vi "2_06.vi"() -> ()   [LabVIEW 2018]
uses:
  <vilib>/sound2/lvsound2.llb/Sound Data Format.ctl
  <vilib>/sound2/lvsound2.llb/Sound Input Read (DBL).vi
  <vilib>/measure/NI_MABase.lvlib
panel:
  out "Meter":dbl(knob) scale=0.0..0.1
  in  "Frecuencia":dbl=10.0 format="%0.2p"
  in  "Longitud de Correlación":dbl=5000.0
  in  "stop":bool
  # "La sensibilidad del correlador a una frecuencia de 440Hz fue un tono 431Hz"
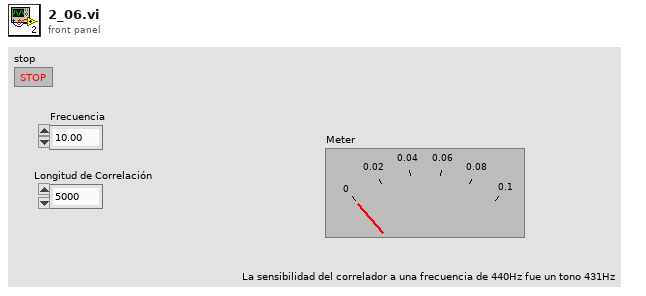
[diagram p1: front panel]
types:
  T1 = typedef "Sound Data Format.ctl" = cluster{"sample rate (S/s)":dbl, "number of channels":i32, "bits per sample":i32}
  T2 = typedef "Sound Input Task ID.ctl" = u32
  T3 = cluster{"sample rate (S/s)":dbl, "Longitud de Correlación":dbl}
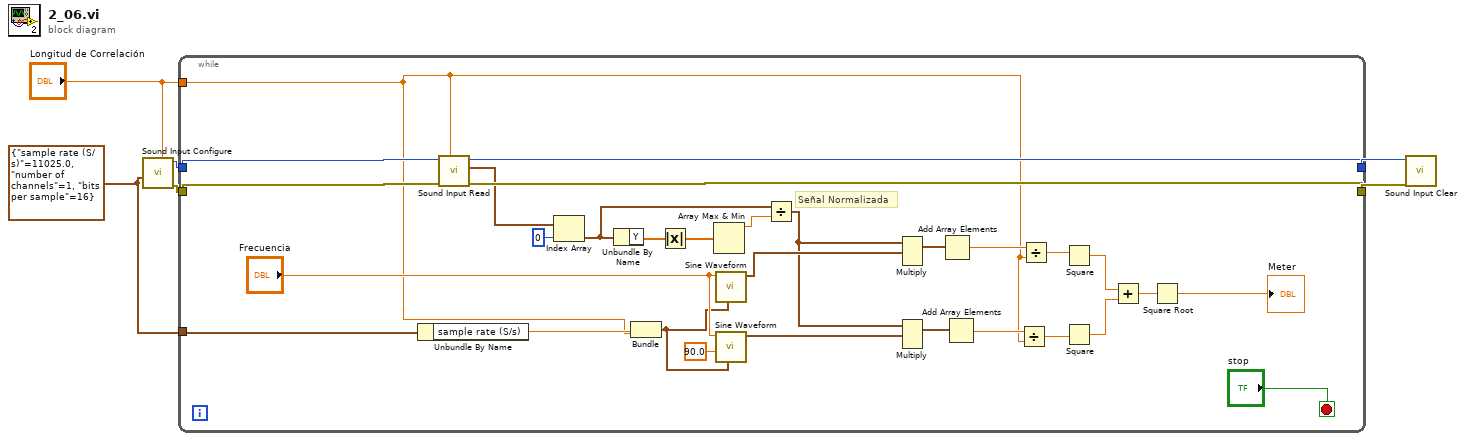
[diagram p0: block diagram]
diagram:
  w1 = T1 {"sample rate (S/s)"=11025.0, "number of channels"=1, "bits per sample"=16} ("sound format")
  n1 = call <vilib>:"Sound Input Configure.vi"("number of samples/ch"="Longitud de Correlación", "sound format"=w1) -> ("error out"=w5:errorcluster, "task ID"=w6:T2)  [unwired: 8 in]
  n2 = while {
    tunnel: w6 -> [w35]
    tunnel: w5 -> [w34]
    tunnel: [w33] -> w4
    tunnel: [w32] -> w3
    tunnel: "Longitud de Correlación" -> [w13]
    tunnel: w1 -> [w24]
    stop <- "stop" stop-if-true
    # "Señal Normalizada"
    n3 = Unbundle By Name(w24) -> ("sample rate (S/s)"=w23:dbl)
    n4 = call-poly <vilib>:"Sound Input Read.vi"("number of samples/ch"=w13, "error in (no error)"=w34, "task ID"=w35) -> ("error out"=w33:errorcluster, "data"=w31:waveform(dbl)[], "task ID out"=w32:T2)  [unwired: 6 in]
    n5 = Index Array(array=w31, index=0) -> (element=w20:waveform(dbl))
    n6 = Unbundle By Name(w20) -> ("Y"=w28:dbl[])
    n7 = Bundle("sample rate (S/s)"=w23, "Longitud de Correlación"=w13) -> (w22:T3)  [unwired: 1 in]
    n8 = Absolute Value(x=w28) -> (abs(x)=w29:dbl[])
    n9 = Array Max & Min(array=w29) -> (max value=w27:dbl)  [unwired: 3 out]
    n10 = call <vilib>:"Sine Waveform.vi"("sampling info"=w22, "frequency"="Frecuencia") -> ("signal out"=w21:waveform(dbl))  [unwired: 8 in, 1 out]
    n11 = call <vilib>:"Sine Waveform.vi"("sampling info"=w22, "phase"=90.0, "frequency"="Frecuencia") -> ("signal out"=w17:waveform(dbl))  [unwired: 7 in, 1 out]
    n12 = Divide(x=w20, y=w27) -> (x/y=w18:waveform(dbl))
    n13 = Multiply(1:w21, 2:w18) -> (0:w19:waveform(dbl))  [unwired: 1 in, 1 out]
    n14 = Multiply(1:w17, 2:w18) -> (0:w16:waveform(dbl))  [unwired: 1 in, 1 out]
    n15 = Add Array Elements(numeric array=w19) -> (sum=w15:dbl)
    n16 = Add Array Elements(numeric array=w16) -> (sum=w14:dbl)
    n17 = Divide(x=w14, y=w13) -> (x/y=w10:dbl)
    n18 = Divide(x=w15, y=w13) -> (x/y=w11:dbl)
    n19 = Square(x=w11) -> (x^2=w9:dbl)
    n20 = Square(x=w10) -> (x^2=w8:dbl)
    n21 = Add(x=w9, y=w8) -> (x+y=w12:dbl)
    n22 = Square Root(x=w12) -> (sqrt(x)=→"Meter":dbl)
  }
  n23 = call <vilib>:"Sound Input Clear.vi"("error in (no error)"=w4, "task ID"=w3) -> ()  [unwired: 9 in, 1 out]
